vi "Configure_Var2.vi"(11 "SMU Config":T1) -> (2 "Vname":string, 3 "Execute?":bool)   [LabVIEW 2012]
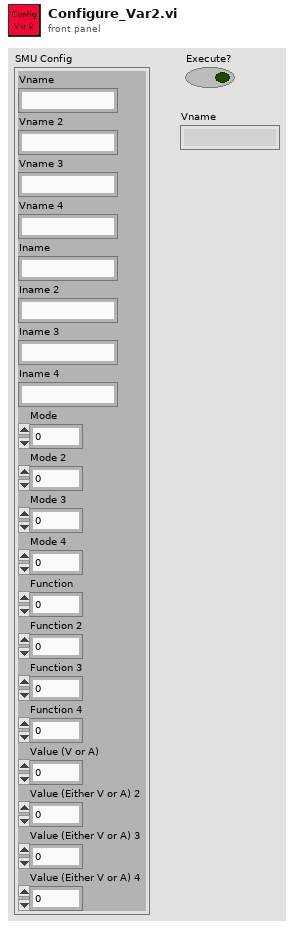
[diagram p1: front panel]
types:
  T1 = cluster{"Vname":string, "Vname 2":string, "Vname 3":string, "Vname 4":string, "Iname":string, "Iname 2":string, "Iname 3":string, "Iname 4":string, "Mode":u16, "Mode 2":u16, "Mode 3":u16, "Mode 4":u16, "Function":u16, "Function 2":u16, "Function 3":u16, "Function 4":u16, "Value (V or A)":dbl, "Value (Either V or A) 2":dbl, "Value (Either V or A) 3":dbl, "Value (Either V or A) 4":dbl}
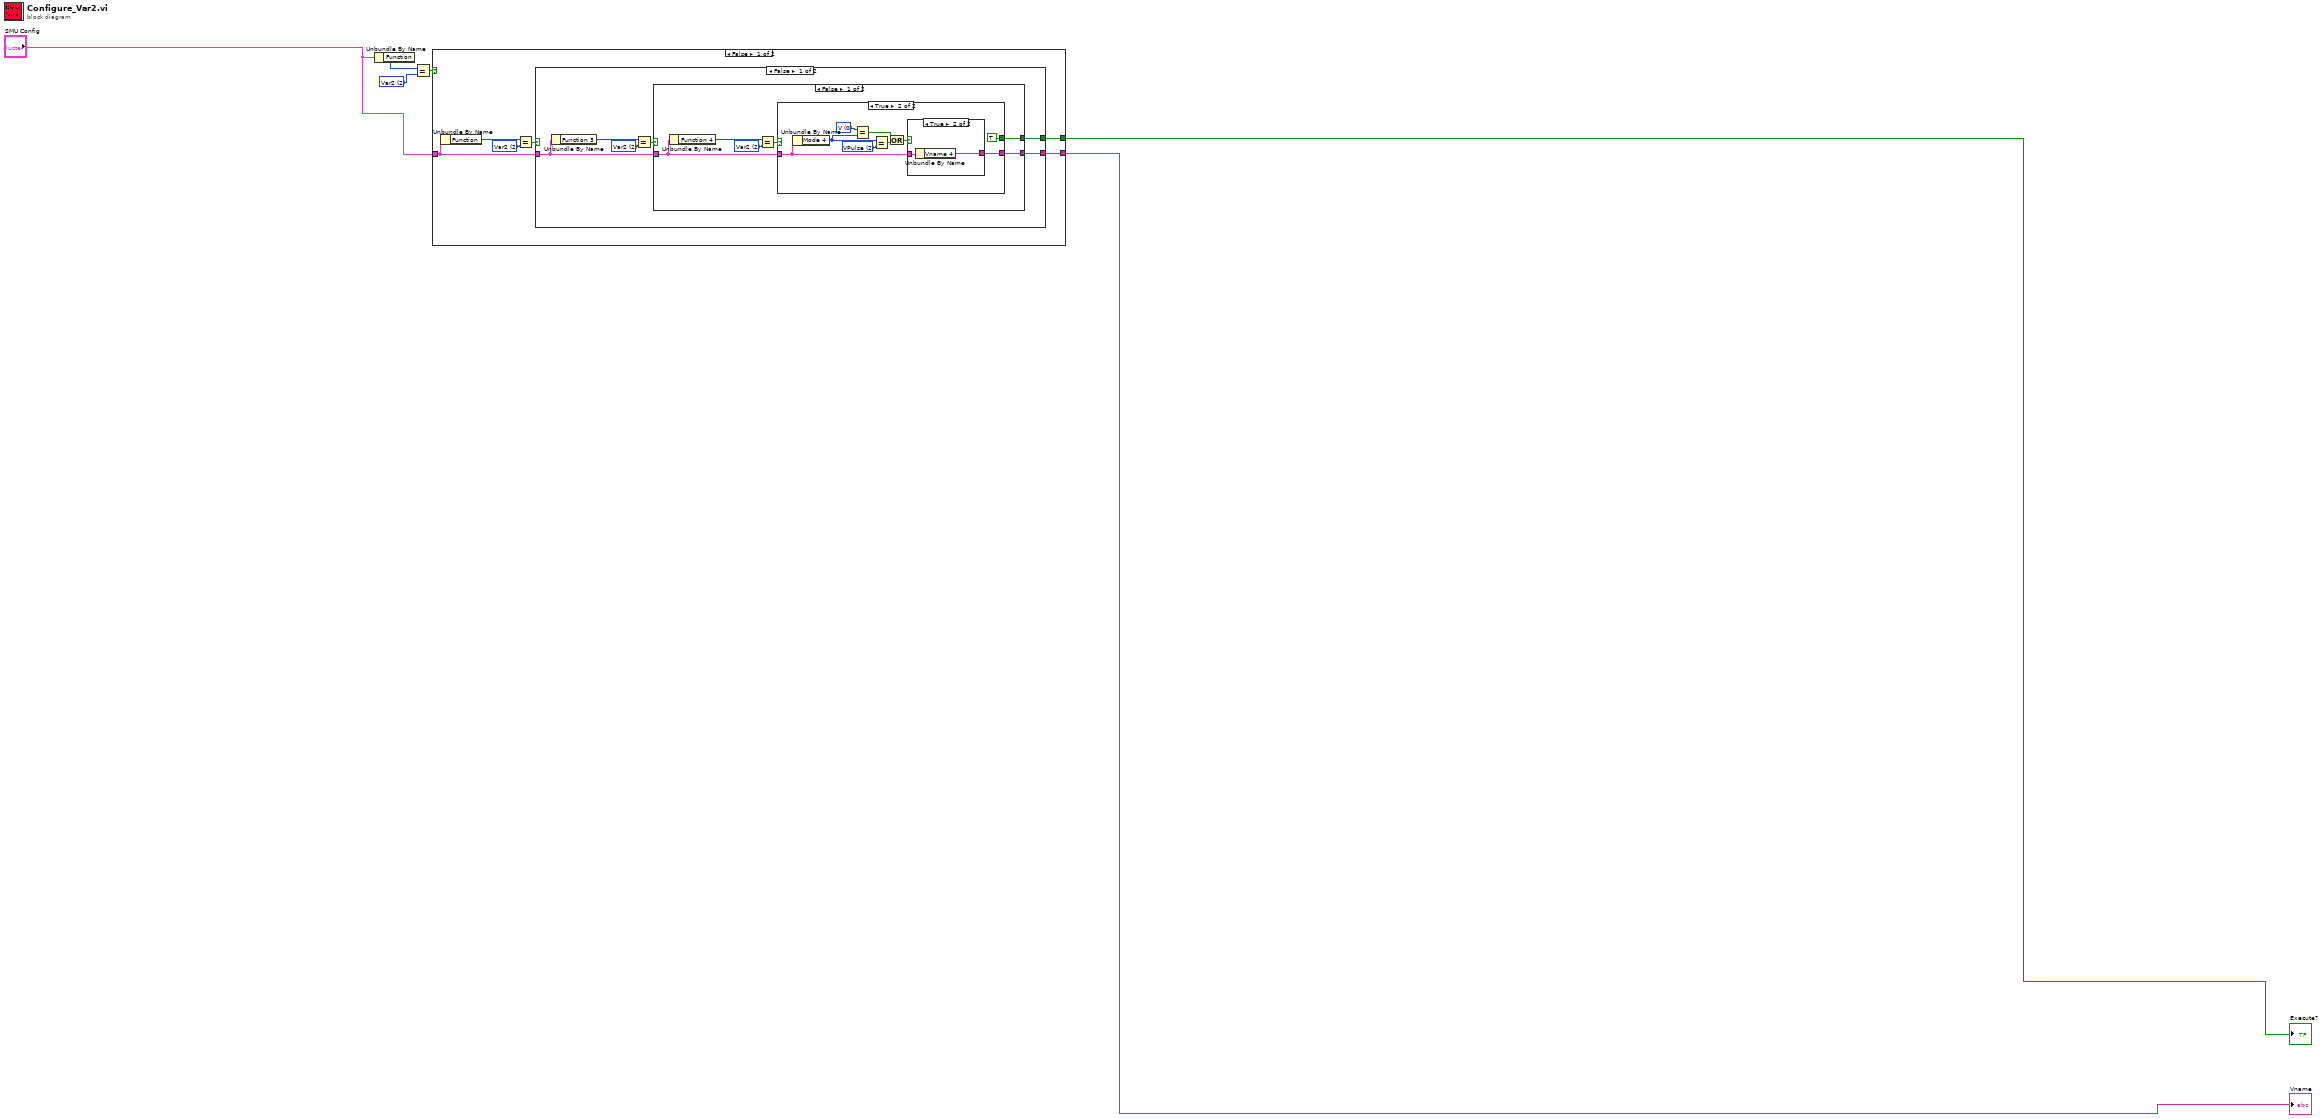
[diagram p0: block diagram]
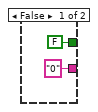
[diagram p2: hidden frame]
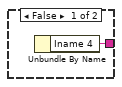
[diagram p3: hidden frame]
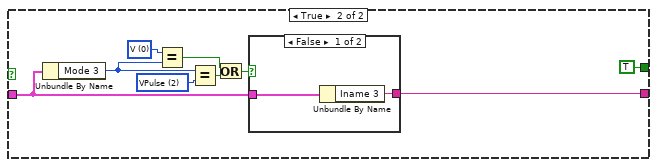
[diagram p4: hidden frame]
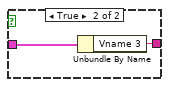
[diagram p5: hidden frame]
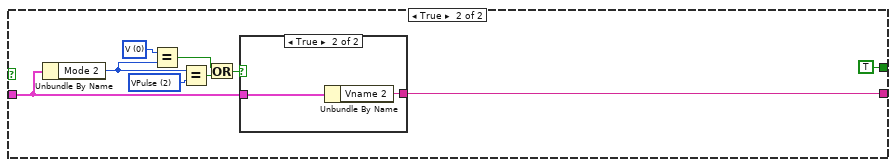
[diagram p6: hidden frame]
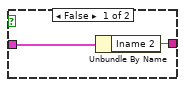
[diagram p7: hidden frame]
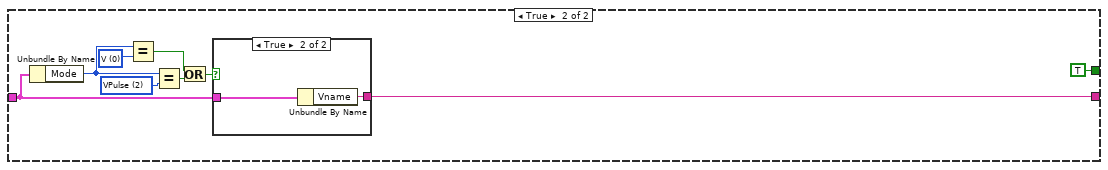
[diagram p8: hidden frame]
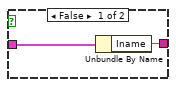
[diagram p9: hidden frame]
diagram:
  w1 = u16 2 items=["disabled", "Var1", "Var2", "Var1'", "Constant"] ("Function")
  n1 = Unbundle By Name("SMU Config") -> ("Function"=w5:u16)
  n2 = Equal?(x=w5, y=w1) -> (x = y?=w2:bool)
  n3 = case shown="False" w2 {
    tunnel: [w10 w73] -> w3
    tunnel: [w9 TRUE ("x = y?")] -> w4
    tunnel: "SMU Config" -> [w8 w65]
    frame False {
      w12 = u16 2 items=["disabled", "Var1", "Var2", "Var1'", "Constant"] ("Function")
      n4 = Unbundle By Name(w8) -> ("Function"=w7:u16)
      n5 = Equal?(x=w7, y=w12) -> (x = y?=w11:bool)
      n6 = case shown="False" w11 {
        tunnel: [w16 w60] -> w10
        tunnel: [w15 TRUE ("x = y?")] -> w9
        tunnel: w8 -> [w14 w53]
        frame False {
          w18 = u16 2 items=["disabled", "Var1", "Var2", "Var1'", "Constant"] ("Function")
          n7 = Unbundle By Name(w14) -> ("Function 3"=w13:u16)
          n8 = Equal?(x=w13, y=w18) -> (x = y?=w17:bool)
          n9 = case shown="False" w17 {
            tunnel: [w24 w47] -> w16
            tunnel: [w21 TRUE ("x = y?")] -> w15
            tunnel: w14 -> [w20 w39]
            frame False {
              w23 = u16 2 items=["disabled", "Var1", "Var2", "Var1'", "Constant"] ("Function")
              n10 = Unbundle By Name(w20) -> ("Function 4"=w19:u16)
              n11 = Equal?(x=w19, y=w23) -> (x = y?=w22:bool)
              n12 = case shown="True" w22 {
                tunnel: ["0" ("Vname 4") w35] -> w24
                tunnel: [FALSE ("x = y?") TRUE ("x = y?")] -> w21
                tunnel: w20 -> [_ w28]
                frame False {
                }
                frame True {
                  w30 = u16 2 items=["V", "I", "VPulse", "IPulse", "Common"] ("Mode 2")
                  w32 = u16 0 items=["V", "I", "VPulse", "IPulse", "Common"] ("Mode 2")
                  n13 = Unbundle By Name(w28) -> ("Mode 4"=w27:u16)
                  n14 = Equal?(x=w32, y=w27) -> (x = y?=w33:bool)
                  n15 = Equal?(x=w27, y=w30) -> (x = y?=w31:bool)
                  n16 = Or(x=w33, y=w31) -> (x .or. y?=w29:bool)
                  n17 = case shown="True" w29 {
                    tunnel: [w36 w37] -> w35
                    tunnel: w28 -> [_ w38]
                    frame False {
                      n18 = Unbundle By Name() -> ("Iname 4"=w36:string)  [unwired: 1 in]
                    }
                    frame True {
                      n19 = Unbundle By Name(w38) -> ("Vname 4"=w37:string)
                    }
                  }
                }
              }
            }
            frame True {
              w43 = u16 2 items=["V", "I", "VPulse", "IPulse", "Common"] ("Mode 2")
              w42 = u16 0 items=["V", "I", "VPulse", "IPulse", "Common"] ("Mode 2")
              n20 = Unbundle By Name(w39) -> ("Mode 3"=w40:u16)
              n21 = Equal?(x=w42, y=w40) -> (x = y?=w45:bool)
              n22 = Equal?(x=w40, y=w43) -> (x = y?=w44:bool)
              n23 = Or(x=w45, y=w44) -> (x .or. y?=w41:bool)
              n24 = case shown="False" w41 {
                tunnel: [w48 w50] -> w47
                tunnel: w39 -> [w49 w51]
                frame False {
                  n25 = Unbundle By Name(w49) -> ("Iname 3"=w48:string)
                }
                frame True {
                  n26 = Unbundle By Name(w51) -> ("Vname 3"=w50:string)
                }
              }
            }
          }
        }
        frame True {
          w55 = u16 2 items=["V", "I", "VPulse", "IPulse", "Common"] ("Mode 2")
          w56 = u16 0 items=["V", "I", "VPulse", "IPulse", "Common"] ("Mode 2")
          n27 = Unbundle By Name(w53) -> ("Mode 2"=w52:u16)
          n28 = Equal?(x=w56, y=w52) -> (x = y?=w58:bool)
          n29 = Equal?(x=w52, y=w55) -> (x = y?=w57:bool)
          n30 = Or(x=w58, y=w57) -> (x .or. y?=w54:bool)
          n31 = case shown="True" w54 {
            tunnel: [w61 w63] -> w60
            tunnel: w53 -> [w62 w64]
            frame False {
              n32 = Unbundle By Name(w62) -> ("Iname 2"=w61:string)
            }
            frame True {
              n33 = Unbundle By Name(w64) -> ("Vname 2"=w63:string)
            }
          }
        }
      }
    }
    frame True {
      w70 = u16 2 items=["V", "I", "VPulse", "IPulse", "Common"] ("Mode")
      w71 = u16 0 items=["V", "I", "VPulse", "IPulse", "Common"] ("Mode")
      n34 = Unbundle By Name(w65) -> ("Mode"=w66:u16)
      n35 = Equal?(x=w66, y=w71) -> (x = y?=w69:bool)
      n36 = Equal?(x=w66, y=w70) -> (x = y?=w68:bool)
      n37 = Or(x=w69, y=w68) -> (x .or. y?=w67:bool)
      n38 = case shown="True" w67 {
        tunnel: [w74 w76] -> w73
        tunnel: w65 -> [w75 w77]
        frame False {
          n39 = Unbundle By Name(w75) -> ("Iname"=w74:string)
        }
        frame True {
          n40 = Unbundle By Name(w77) -> ("Vname"=w76:string)
        }
      }
    }
  }
  "Execute?" <- w4
  "Vname" <- w3
